vi "Add Athlete Dialogue.vi"(0 "Enable":bool=TRUE, 1 "Name":T1, 5 "error in (no error)":errorcluster) -> (16 "Team":string, 17 "Athlete":string, 18 "OK":bool, 19 "error out":errorcluster)   [LabVIEW 2020]
doc: "Displays a standard dialog box that prompts users to enter information, such as a user name and password.\n--------------------\n\nThis Express VI is configured as follows:\n\nMessage to Display to the User:Add User\nThe inputs are: \nText Entry Box: Athlete\nText Entry Box: Team"
uses:
  Name--cluster.ctl
  Data Manager.lvclass
panel:
  in  "Team":string="Unknown"
  in  "Athlete":string="Unknown"
  out "String":string="Add Athlete to Database"
  in  "Cancel":bool
  in  "OK2":bool
  in  "OK1":bool
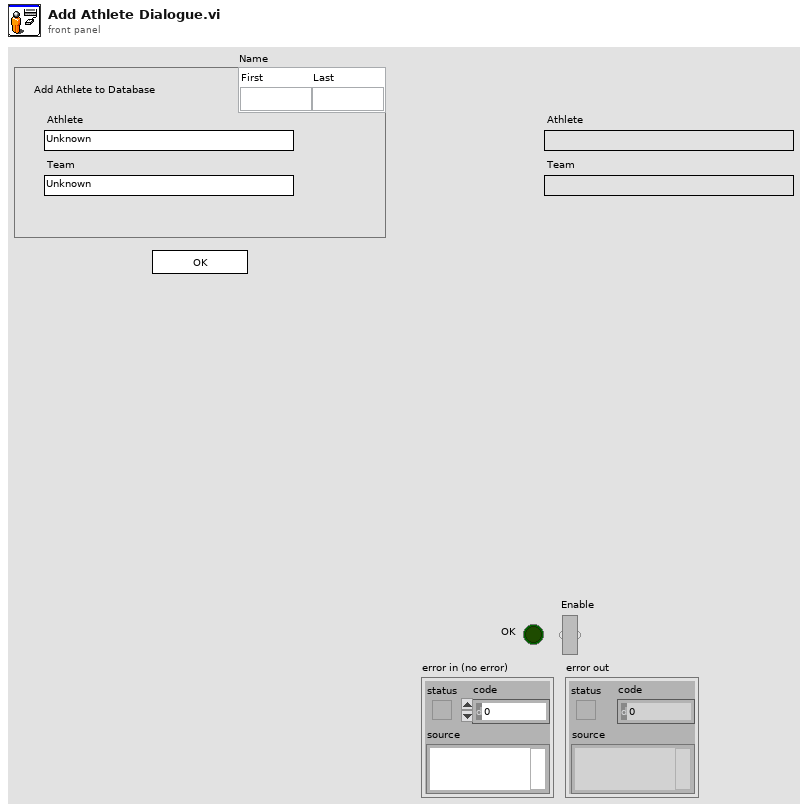
[diagram p1: front panel]
types:
  T1 = typedef "Data Manager.lvclass/Name--cluster.ctl" = cluster{"First":string, "Last":string}
  T2 = cluster{"Input Name":string, "Input Data Type":i32}[]
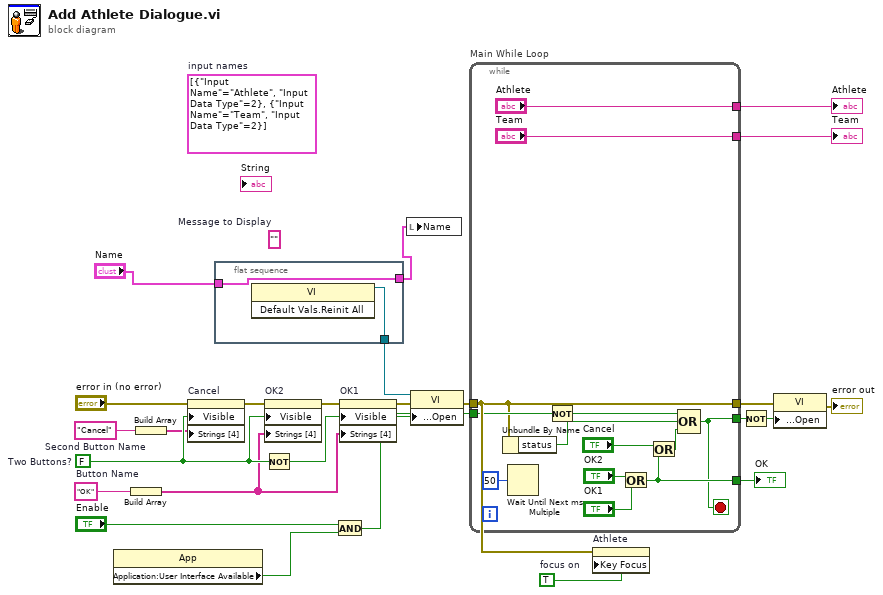
[diagram p0: block diagram]
diagram:
  w4 = TRUE  # focus on
  (unwired) T2 [{"Input Name"="Athlete", "Input Data Type"=2}, {"Input Name"="Team", "Input Data Type"=2}]  # input names
  w17 = "Cancel"  # Second Button Name
  w15 = "OK"  # Button Name
  (unwired) ""  # Message to Display
  w25 = FALSE  # Two Buttons?
  n1 = property class="App"() -> ("Application:User Interface Available"=w7:bool)  [unwired: 2 in, 2 out]
  n2 = Build Array(w15) -> (w16:string[])
  n3 = Build Array(w17) -> (w18:string[])
  n4 = property on="Cancel" class="Bool"(error in="error in (no error)", "Visible"=w25, "Strings [4]"=w18) -> (error out=w22:errorcluster)  [unwired: 1 in, 1 out]
  n5 = flat-sequence {
    tunnel: [w27] -> w6
    tunnel: [w26] -> w1
    tunnel: "Name" -> [w26]
    frame #0 {
      n6 = invoke class="VI" method="Default Vals.Reinit All"() -> (reference out=w27:refnum<vi>)  [unwired: 3 in, 2 out]
    }
  }
  n7 = Not(x=w25) -> (.not. x?=w23:bool)
  n8 = property on="OK2" class="Bool"(error in=w22, "Visible"=w25, "Strings [4]"=w16) -> (error out=w21:errorcluster)  [unwired: 1 in, 1 out]
  n9 = And(x="Enable", y=w7) -> (x .and. y?=w8:bool)
  n10 = property on="OK1" class="Bool"(error in=w21, "Visible"=w23, "Strings [4]"=w16) -> (error out=w14:errorcluster)  [unwired: 1 in, 1 out]
  n11 = local write "Name"(w1) -> ()
  n12 = property class="VI"(reference=w6, error in=w14, "Front Panel Window:Open"=w8) -> (error out=w13:errorcluster)  [unwired: 1 out]
  n13 = while "Main While Loop" {
    tunnel: [w37] -> w24
    tunnel: w8 -> [w35]
    tunnel: [w33] -> w19
    tunnel: w13 -> [w32]
    tunnel: [w32] -> w11
    tunnel: ["Athlete"] -> w5
    tunnel: ["Team"] -> w3
    stop <- w33 stop-if-true
    n14 = Unbundle By Name(w32) -> ("status"=w30:bool)
    n15 = Wait Until Next ms Multiple(millisecond multiple=u32 50) -> ()  [unwired: 1 out]
    n16 = Not(x=w35) -> (.not. x?=w34:bool)
    n17 = Or(x="OK2", y="OK1") -> (x .or. y?=w37:bool)
    n18 = Or(x="Cancel", y=w37) -> (x .or. y?=w31:bool)
    n19 = Compound Arithmetic op=OR(w34, w30, w31) -> (w33:bool)
  }
  "OK" <- w24
  "Athlete" <- w5
  "Team" <- w3
  n20 = property on="Athlete" class="Str"(error in=w13, "Key Focus"=w4) -> ()  [unwired: 1 in, 2 out]
  n21 = Not(x=w19) -> (.not. x?=w20:bool)
  n22 = property class="VI"(error in=w11, "Front Panel Window:Open"=w20) -> (error out=→"error out":errorcluster)  [unwired: 1 in, 1 out]
